vi "Point Data Updated.vi"(8 "error in":errorcluster, 9 "Data":variant, 10 "Task-Point Ident":string, 11 "Series UI Actor in":refnum<class "Series UI Actor.lvclass">) -> (0 "error out":errorcluster, 3 "Series UI Actor out":refnum<class "Series UI Actor.lvclass">)   [LabVIEW 2024, in "Series UI Actor.lvlib" / "Series UI Actor.lvclass"]
uses:
  Series UI Actor.lvclass
  Series UI Actor.lvclass/Series UI Actor.ctl
  <vilib>/Utility/miscctls.llb/LVMapReplaceAction.ctl
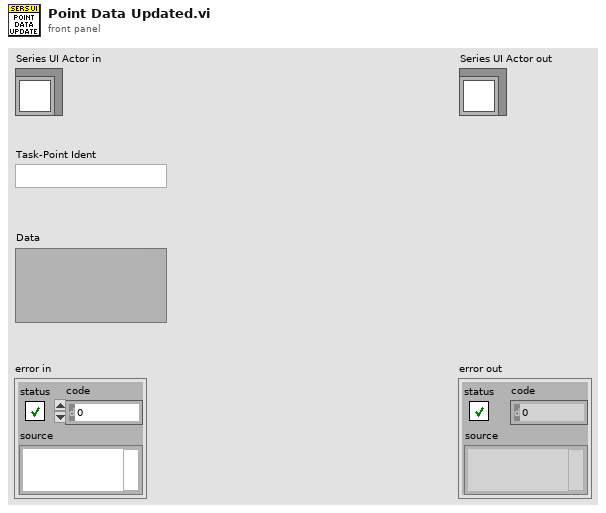
[diagram p1: front panel]
types:
  T1 = typedef "LVMapReplaceAction.ctl" = enum32{"Modify Entry only if found", "Add or Modify Entry", "Delete Entry"}
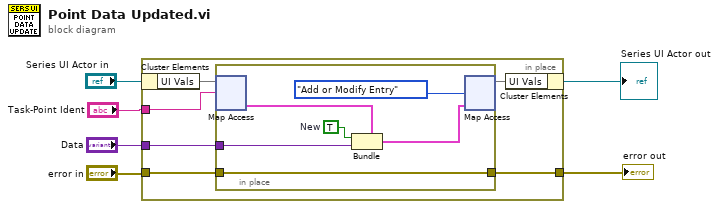
[diagram p0: block diagram]
diagram:
  n1 = in-place {
    in-place-border: "Task-Point Ident" -> [w7]
    in-place-border: "error in" -> [w11]
    in-place-border: "Data" -> [w10]
    in-place-border: [w9] -> w1
    n2 = in-place-cluster #1("Series UI Actor in") -> ("UI Vals"=w12:map{string, cluster{"New?":bool, variant}})
    n3 = in-place {
      in-place-border: w11 -> [w18]
      in-place-border: w10 -> [w15]
      in-place-border: [w18] -> w9
      w16 = TRUE  # New
      n4 = in-place-map #2(w12, w7) -> (w13:cluster{"New?":bool, variant})  [unwired: 1 in, 1 out]
      n5 = Bundle(cluster=w13, "New?"=w16, w15) -> (w14:cluster{"New?":bool, variant})
      n6 = in-place-map #2(w14, LVMapReplaceAction."Add or Modify Entry" ("action")) -> (w8:map{string, cluster{"New?":bool, variant}})  [unwired: 2 out]
    }
    n7 = in-place-cluster #1("UI Vals"=w8) -> (→"Series UI Actor out":refnum<class "Series UI Actor.lvclass">)
  }
  "error out" <- w1
